vi "IsNewHighscore.vi"(8 "error in (no error)":errorcluster, 10 "Score":dbl, 11 "Highscore in":refnum<class "Highscore.lvclass">) -> (0 "error out":errorcluster, 2 "IsNewHighscore?":bool, 3 "Highscore out":refnum<class "Highscore.lvclass">)   [LabVIEW 2019, in "RT_Game.lvlib" / "Highscore.lvclass"]
uses:
  Highscore.lvclass
  Highscore.lvclass/Highscore.ctl
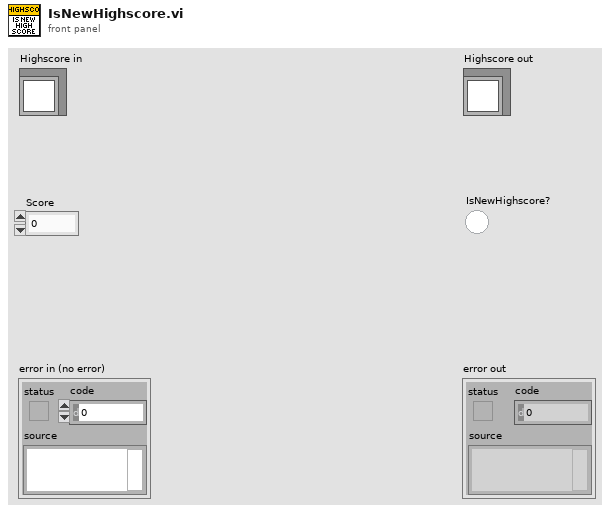
[diagram p1: front panel]
types:
  T1 = typedef "RT_Game.lvlib/Highscore.lvclass/HighscoreEntry.ctl" = cluster{"Name":string, "Score":dbl}
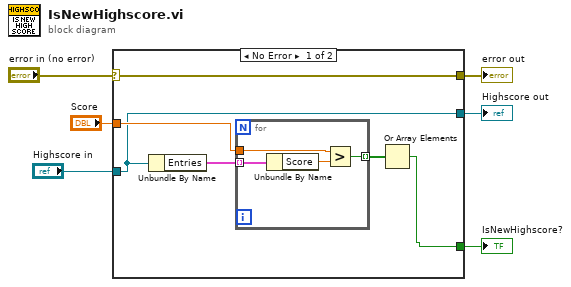
[diagram p0: block diagram]
diagram:
  n1 = case shown="No Error" "error in (no error)" {
    selector: "error in (no error)" -> [w12 w18]
    tunnel: [w12 w18] -> w5
    tunnel: [w8 w17] -> w3
    tunnel: "Highscore in" -> [w8 w17]
    tunnel: "Score" -> [w10 _]
    tunnel: [w7 _] -> w1
    frame No Error {
      n2 = Unbundle By Name(w8) -> ("Entries"=w11:T1[])
      n3 = for {
        tunnel: w11 -> [w16] mode=indexing
        tunnel: w10 -> [w15]
        tunnel: [w13] -> w9 mode=indexing
        n4 = Unbundle By Name(w16) -> ("Score"=w14:dbl)
        n5 = Greater?(x=w15, y=w14) -> (0:w13:bool)
      }
      n6 = Or Array Elements(Boolean array=w9) -> (logical OR=w7:bool)
    }
    frame Error {
    }
  }
  "error out" <- w5
  "Highscore out" <- w3
  "IsNewHighscore?" <- w1
